vi "G_Estados_Desmenuzadora.vi"() -> ()   [LabVIEW 2020]
panel:
  out "Estados_Desmenuzadora":cluster{"Desmenuzadora":bool, "Aspa":bool}
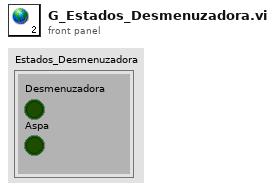
[diagram p1: front panel]
diagram:
